vi "CreateLogger.vi"(8 "error in (no error)":errorcluster, 9 "Name":string, 10 "ModulePath":path, 11 "Logger in":refnum<class "Logger.lvclass">) -> (0 "error out":errorcluster, 3 "Logger out":refnum<class "Logger.lvclass">)   [LabVIEW 2022 SP3, in "Logger.lvlib" / "Logger.lvclass"]
uses:
  Logger.lvclass
  C:/Users/jakub/repos/gh/PythonWrapper/Source/PythonWrapper/PythonWrapper.lvclass
  PythonWrapper/Source/PythonWrapper/PythonWrapper.lvclass/PythonWrapper.ctl
  Logger.lvclass/Logger.ctl
  PythonWrapper/Source/PythonWrapper/Read PythonSession.vi
  PythonWrapper/Source/PythonWrapper/Read ModulePath.vi
  Read Logger.vi
  Write Logger.vi
  Write Name.vi
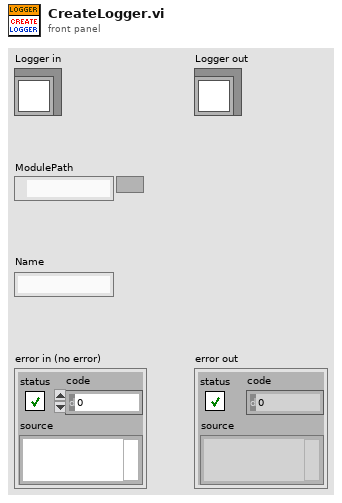
[diagram p1: front panel]
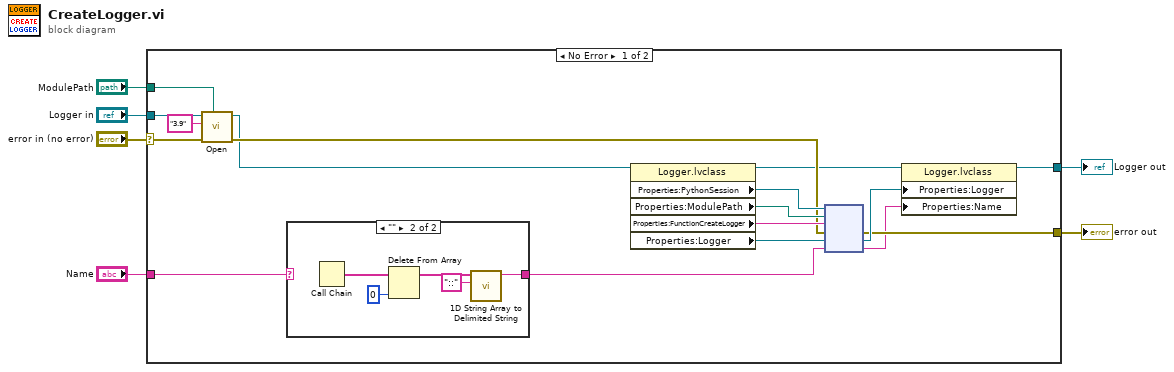
[diagram p0: block diagram]
diagram:
  n1 = case shown="No Error" "error in (no error)" {
    selector: "error in (no error)" -> [w23 w31]
    tunnel: [w10 w31] -> w5
    tunnel: [w11 w30] -> w3
    tunnel: "Logger in" -> [w20 w30]
    tunnel: "Name" -> [w8 _]
    tunnel: "ModulePath" -> [w21 _]
    frame No Error {
      n2 = call-dynamic "Open.vi"("ModulePath"=w21, "error in (no error)"=w23, "PythonVersion"="3.9", "PythonWrapper in"=w20) -> ("error out"=w16:errorcluster, "PythonWrapper out"=w12:refnum<class "Logger.lvclass">)  [unwired: 6 in]
      n3 = case shown="\"\"" w8 {
        selector: w8 -> [w24 _]
        tunnel: [w24 w28] -> w9
        frame Default {
        }
        frame "" {
          n4 = Call Chain() -> (call chain=w27:string[])
          n5 = Delete From Array(array=w27, index=0) -> (array with subset deleted=w26:string[])  [unwired: 1 in, 1 out]
          n6 = call <vilib>:"1D String Array to Delimited String.vi"("delimiter"="::", "string array"=w26) -> ("delimited string"=w28:string)  [unwired: 9 in]
        }
      }
      n7 = property class="Logger.lvclass"(reference=w12) -> (reference out=w15:refnum<class "Logger.lvclass">, "Properties:PythonSession"=w19:refnum<k35>, "Properties:ModulePath"=w18:path, "Properties:FunctionCreateLogger"=w17:string, "Properties:Logger"=w14:refnum<k38>)  [unwired: 1 in, 1 out]
      n8 = node(w19, w18, w17, w16, w14, w9) -> (w10:errorcluster, w13:refnum<k38>, w7:string)  [unwired: 3 out]
      n9 = property class="Logger.lvclass"(reference=w15, "Properties:Logger"=w13, "Properties:Name"=w7) -> (reference out=w11:refnum<class "Logger.lvclass">)  [unwired: 1 in, 1 out]
    }
    frame Error {
    }
  }
  "error out" <- w5
  "Logger out" <- w3
